vi "Determine Padding.vi"(8 "error in":errorcluster, 11 "Instruments in":refnum<class "Instruments.lvclass">) -> (0 "error out":errorcluster, 3 "Instruments out":refnum<class "Instruments.lvclass">)   [LabVIEW 2023, in "Instruments.lvlib" / "Instruments.lvclass"]
uses:
  Library/Instruments.lvclass
  Library/Instruments.lvclass/Instruments.ctl
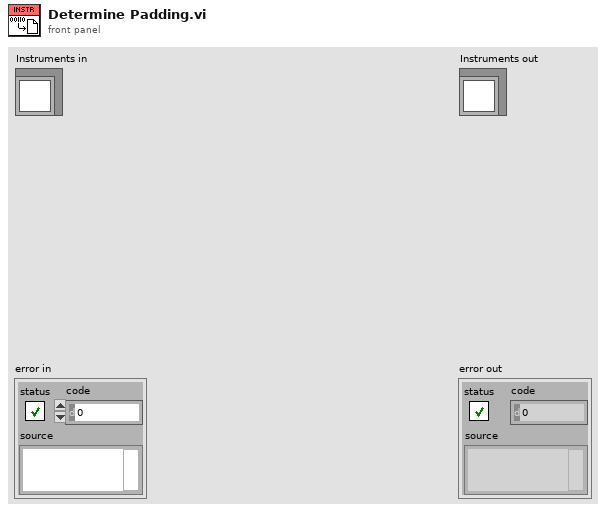
[diagram p1: front panel]
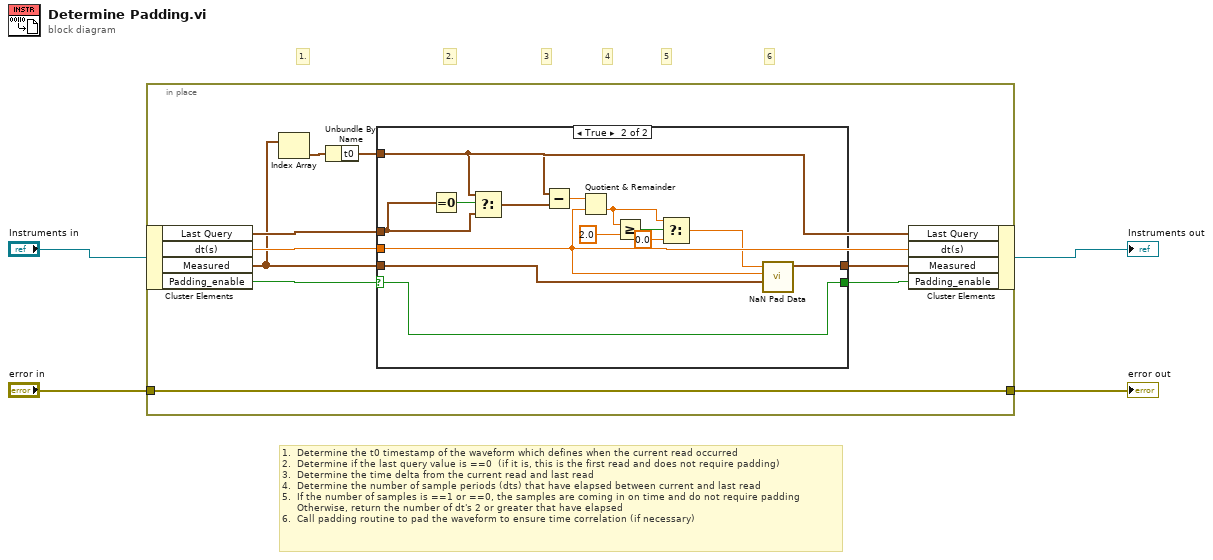
[diagram p0: block diagram]
diagram:
  # "1.  Determine the t0 timestamp of the waveform which defines when the current read occurred\n2.  Determine if the last query value is ==0  (if it is, this is the first read and does not require padding)\n3.  Determine the time delta from the current read and last read\n4.  Determine the number of sample periods (dts) that have elapsed between current and last read\n5.  If the number of samples is ==1 or ==0, the samples are coming in on time and do not require padding\n     Otherwise, return the number of dt's 2 or greater that have elapsed\n6.  Call padding routine to pad the waveform to ensure time correlation (if necessary)"
  # "6"
  # "5"
  # "4"
  # "3"
  # "2."
  # "1."
  n1 = in-place {
    in-place-border: [w12] -> w3
    in-place-border: "error in" -> [w12]
    n2 = in-place-cluster #1("Instruments in") -> ("Last Query"=w11:timestamp, "dt(s)"=w9:dbl, "Measured"=w8:waveform(dbl)[], "Padding_enable"=w6:bool)
    n3 = Index Array(array=w8) -> (element=w7:waveform(dbl))  [unwired: 1 in]
    n4 = Unbundle By Name(w7) -> ("t0"=w10:timestamp)
    n5 = case shown="True" w6 {
      selector: w6 -> [w14 w16]
      tunnel: [w15 w29] -> w13
      tunnel: w11 -> [_ w28]
      tunnel: w10 -> [_ w27]
      tunnel: w9 -> [_ w26]
      tunnel: w8 -> [w15 w25]
      tunnel: [w14 w16] -> w5
      frame False {
      }
      frame True {
        n6 = Equal To 0?(x=w28) -> (x = 0?=w17:bool)
        n7 = Select(t=w27, s=w17, f=w28) -> (s? t:f=w23:timestamp)
        n8 = Subtract(x=w27, y=w23) -> (x-y=w24:dbl)
        n9 = Quotient & Remainder(x=w24, y=w26) -> (floor(x/y)=w20:dbl)  [unwired: 1 out]
        n10 = Greater Or Equal?(x=w20, y=2.0) -> (x >= y?=w21:bool)
        n11 = Select(t=w20, s=w21, f=0.0) -> (s? t:f=w18:dbl)
        n12 = call "NaN Pad Data.vi"("Measured"=w25, "dt(s)"=w26, "Num dts elapsed"=w18) -> ("Array"=w29:waveform(dbl)[])  [unwired: 8 in]
      }
    }
    n13 = in-place-cluster #1("Last Query"=w10, "dt(s)"=w9, "Measured"=w13, "Padding_enable"=w5) -> (→"Instruments out":refnum<class "Instruments.lvclass">)
  }
  "error out" <- w3
